vi "Has Value.vi"(11 "Entity in":refnum<class "Entity.lvclass">) -> (2 "Has Value":bool)   [LabVIEW 2020, in "Conditu2.lvlib" / "Columns.lvlib" / "Entity.lvclass"]
uses:
  Entity.lvclass
  Entity.lvclass/Entity.ctl
  Entity/Entity.lvclass/Entity.ctl
  ID/ID.lvclass/ID.ctl
  ID/Get.vi
  Entity/Entity.lvclass
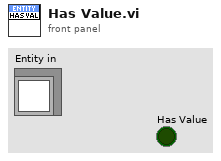
[diagram p1: front panel]
types:
  T1 = typedef "Conditu2.lvlib/Entity ID.ctl" = i64
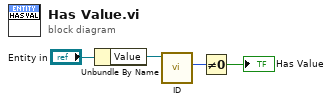
[diagram p0: block diagram]
diagram:
  n1 = Unbundle By Name("Entity in") -> ("Value"=w3:refnum<class "Entity.lvclass">)
  n2 = call "ID.vi"("Entity in"=w3) -> ("ID"=w2:T1)  [unwired: 9 in, 1 out]
  n3 = Not Equal To 0?(x=w2) -> (x != 0?=→"Has Value":bool)
